vi "test.vi"() -> ()   [LabVIEW 2019]
panel:
  out "origin":dbl[](array[numeric])
  out "+1":dbl[](array[numeric])
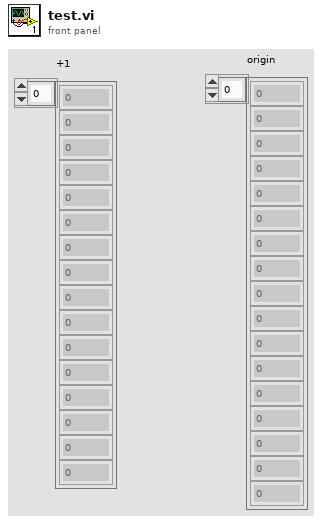
[diagram p1: front panel]
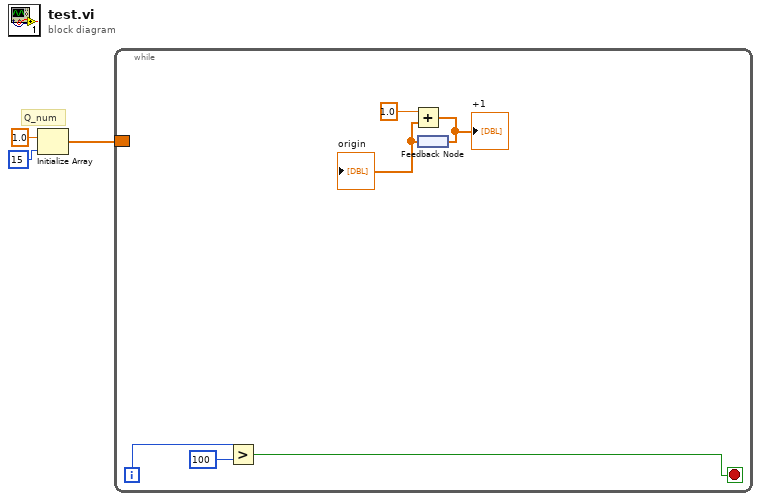
[diagram p0: block diagram]
diagram:
  # "Q_num"
  n1 = Initialize Array(1.0 ("element"), 15 ("dimension size")) -> (w1:dbl[])
  n2 = while {
    border: w1 -> [_]
    i -> [w8]
    stop <- w6 stop-if-true
    n3 = Greater?(x=w8, y=100) -> (0:w6:bool)
    n4 = feedback #1() -> (w9:dbl[])
    "origin" <- w9
    n5 = Add(x=1.0, y=w9) -> (x+y=w4:dbl[])
    "+1" <- w4
    n6 = feedback-in #1(w4) -> ()
  }
